vi "dispose dataset.vi"(8 "error in":errorcluster, 11 "TLS HTTP handler dataset in":refnum<class "TLS HTTP handler dataset.lvclass">) -> (0 "error out":errorcluster)   [LabVIEW 2016, in "TLS HTTP handler dataset.lvclass"]
uses:
  TLS HTTP handler dataset.lvclass
  TLS HTTP handler dataset.lvclass/TLS HTTP handler dataset.ctl
  lvlibtls/server/lvlibretls server listener.lvclass
  HTTP handler dataset/basic HTTP handler dataset.lvclass
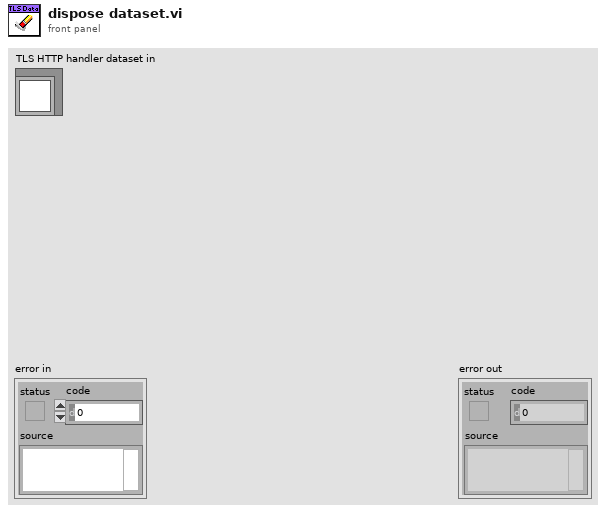
[diagram p1: front panel]
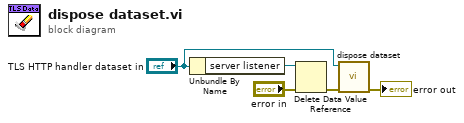
[diagram p0: block diagram]
diagram:
  n1 = Unbundle By Name("TLS HTTP handler dataset in") -> ("server listener"=w1:refnum<data-value>)
  n2 = Delete Data Value Reference(data value reference=w1, error in="error in") -> (error out=w3:errorcluster)  [unwired: 1 out]
  n3 = call-parent "dispose dataset.vi"("error in"=w3, "basic HTTP handler dataset in"="TLS HTTP handler dataset in") -> ("error out"=→"error out":errorcluster)  [unwired: 9 in]
